vi "Build Simple Skeleton Data.vi"(8 "error in (no error)":errorcluster, 11 "connection ID":refnum<k16>) -> (0 "Kinect Outputs":T5, 1 "Skeleton Data":T6, 2 "NumPlayers":i8, 3 "Version String":string, 4 "Simple Joystick Info":T1(array[cluster]))   [LabVIEW 2013]
uses:
  <vilib>/addons/Kinect/SkeletonTrackState.ctl
  <vilib>/addons/Kinect/Vector4.ctl
  <vilib>/Rock Robotics/WPI/Joystick/WPI_JoystickDeviceDataRaw.ctl
  <vilib>/Rock Robotics/WPI/Dashboard/WPI_DashboardLogging Global.vi
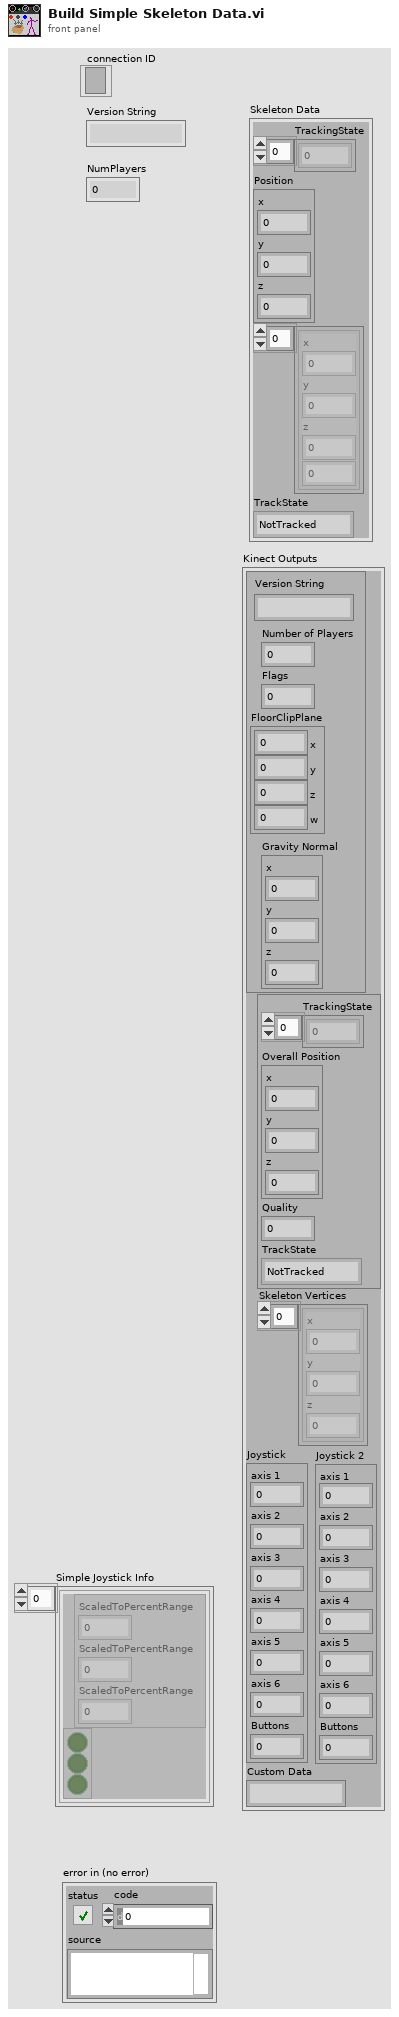
[diagram p1: front panel]
types:
  T1 = cluster{cluster{"ScaledToPercentRange":dbl, "ScaledToPercentRange":dbl, "ScaledToPercentRange":dbl}, cluster{bool, bool, bool}}[]
  T2 = typedef "Vector4.ctl" = cluster{"x":sgl, "y":sgl, "z":sgl, "w":sgl}
  T3 = typedef "SkeletonTrackState.ctl" = enum32{"NotTracked", "PositionOnly", "Tracked"}
  T4 = typedef "WPI_JoystickDeviceDataRaw.ctl" = cluster{"axis 1":i8, "axis 2":i8, "axis 3":i8, "axis 4":i8, "axis 5":i8, "axis 6":i8, "Buttons":u16}
  T5 = cluster{cluster{"Version String":string, "Number of Players":i8, "Flags":u32, "FloorClipPlane":T2, "Gravity Normal":cluster{"x":sgl, "y":sgl, "z":sgl}}, cluster{"TrackingState":u8[], "Overall Position":cluster{"x":sgl, "y":sgl, "z":sgl}, "Quality":u32, "TrackState":T3}, "Skeleton Vertices":cluster{"x":sgl, "y":sgl, "z":sgl}[], "Joystick":T4, "Joystick 2":T4, "Custom Data":string}
  T6 = cluster{"TrackingState":u8[], "Position":cluster{"x":sgl, "y":sgl, "z":sgl}, cluster{"x":sgl, "y":sgl, "z":sgl, sgl}[], "TrackState":T3}
  T7 = cluster{"size":u8, "tag":u8, "Version":cluster{"unsigned byte array[0]":u8, "unsigned byte array[1]":u8, "unsigned byte array[2]":u8, "unsigned byte array[3]":u8, "unsigned byte array[4]":u8, "unsigned byte array[5]":u8, "unsigned byte array[6]":u8, "unsigned byte array[7]":u8, "unsigned byte array[8]":u8, "unsigned byte array[9]":u8, "unsigned byte array[10]":u8}, "numPlayers":i8, "flags":u32, "floorClipPlane":T2, "Gravity Normal":cluster{"x":sgl, "y":sgl, "z":sgl}, "size":u8, "tag":u8, "Extra Data":cluster{"TrackingState":cluster{"TrackingState[0]":u8, "TrackingState[1]":u8, "TrackingState[2]":u8, "TrackingState[3]":u8, "TrackingState[4]":u8, "TrackingState[5]":u8, "TrackingState[6]":u8, "TrackingState[7]":u8, "TrackingState[8]":u8, "TrackingState[9]":u8, "TrackingState[10]":u8, "TrackingState[11]":u8, "TrackingState[12]":u8, "TrackingState[13]":u8, "TrackingState[14]":u8, "TrackingState[15]":u8, "TrackingState[16]":u8, "TrackingState[17]":u8, "TrackingState[18]":u8, "TrackingState[19]":u8}, "Position":cluster{"x":sgl, "y":sgl, "z":sgl}, "Quality":u32, "TrackState":T3}, "size":u8, "tag":u8, "Vertices":cluster{"Vertices[0]":cluster{"x":sgl, "y":sgl, "z":sgl}, "Vertices[1]":cluster{"x":sgl, "y":sgl, "z":sgl}, "Vertices[2]":cluster{"x":sgl, "y":sgl, "z":sgl}, "Vertices[3]":cluster{"x":sgl, "y":sgl, "z":sgl}, "Vertices[4]":cluster{"x":sgl, "y":sgl, "z":sgl}, "Vertices[5]":cluster{"x":sgl, "y":sgl, "z":sgl}, "Vertices[6]":cluster{"x":sgl, "y":sgl, "z":sgl}, "Vertices[7]":cluster{"x":sgl, "y":sgl, "z":sgl}, "Vertices[8]":cluster{"x":sgl, "y":sgl, "z":sgl}, "Vertices[9]":cluster{"x":sgl, "y":sgl, "z":sgl}, "Vertices[10]":cluster{"x":sgl, "y":sgl, "z":sgl}, "Vertices[11]":cluster{"x":sgl, "y":sgl, "z":sgl}, "Vertices[12]":cluster{"x":sgl, "y":sgl, "z":sgl}, "Vertices[13]":cluster{"x":sgl, "y":sgl, "z":sgl}, "Vertices[14]":cluster{"x":sgl, "y":sgl, "z":sgl}, "Vertices[15]":cluster{"x":sgl, "y":sgl, "z":sgl}, "Vertices[16]":cluster{"x":sgl, "y":sgl, "z":sgl}, "Vertices[17]":cluster{"x":sgl, "y":sgl, "z":sgl}, "Vertices[18]":cluster{"x":sgl, "y":sgl, "z":sgl}, "Vertices[19]":cluster{"x":sgl, "y":sgl, "z":sgl}}, "size":u8, "tag":u8, "Joystick":T4, "Joystick 2":T4, "size":u8, "tag":u8, "Custom Data":string}
  T8 = cluster{"size":u8, "tag":u8, "Version":cluster{"unsigned byte array[0]":u8, "unsigned byte array[1]":u8, "unsigned byte array[2]":u8, "unsigned byte array[3]":u8, "unsigned byte array[4]":u8, "unsigned byte array[5]":u8, "unsigned byte array[6]":u8, "unsigned byte array[7]":u8, "unsigned byte array[8]":u8, "unsigned byte array[9]":u8, "unsigned byte array[10]":u8}, "numPlayers":i8, "flags":u32, "floorClipPlane":T2, "Gravity Normal":cluster{"x":sgl, "y":sgl, "z":sgl}, "size":u8, "tag":u8, "Extra Data":cluster{"TrackingState":cluster{"TrackingState[0]":u8, "TrackingState[1]":u8, "TrackingState[2]":u8, "TrackingState[3]":u8, "TrackingState[4]":u8, "TrackingState[5]":u8, "TrackingState[6]":u8, "TrackingState[7]":u8, "TrackingState[8]":u8, "TrackingState[9]":u8, "TrackingState[10]":u8, "TrackingState[11]":u8, "TrackingState[12]":u8, "TrackingState[13]":u8, "TrackingState[14]":u8, "TrackingState[15]":u8, "TrackingState[16]":u8, "TrackingState[17]":u8, "TrackingState[18]":u8, "TrackingState[19]":u8}, "Position":cluster{"x":sgl, "y":sgl, "z":sgl}, "Quality":u32, "TrackState":T3}, "size":u8, "tag":u8, "Vertices":cluster{"Vertices[0]":cluster{"x":sgl, "y":sgl, "z":sgl}, "Vertices[1]":cluster{"x":sgl, "y":sgl, "z":sgl}, "Vertices[2]":cluster{"x":sgl, "y":sgl, "z":sgl}, "Vertices[3]":cluster{"x":sgl, "y":sgl, "z":sgl}, "Vertices[4]":cluster{"x":sgl, "y":sgl, "z":sgl}, "Vertices[5]":cluster{"x":sgl, "y":sgl, "z":sgl}, "Vertices[6]":cluster{"x":sgl, "y":sgl, "z":sgl}, "Vertices[7]":cluster{"x":sgl, "y":sgl, "z":sgl}, "Vertices[8]":cluster{"x":sgl, "y":sgl, "z":sgl}, "Vertices[9]":cluster{"x":sgl, "y":sgl, "z":sgl}, "Vertices[10]":cluster{"x":sgl, "y":sgl, "z":sgl}, "Vertices[11]":cluster{"x":sgl, "y":sgl, "z":sgl}, "Vertices[12]":cluster{"x":sgl, "y":sgl, "z":sgl}, "Vertices[13]":cluster{"x":sgl, "y":sgl, "z":sgl}, "Vertices[14]":cluster{"x":sgl, "y":sgl, "z":sgl}, "Vertices[15]":cluster{"x":sgl, "y":sgl, "z":sgl}, "Vertices[16]":cluster{"x":sgl, "y":sgl, "z":sgl}, "Vertices[17]":cluster{"x":sgl, "y":sgl, "z":sgl}, "Vertices[18]":cluster{"x":sgl, "y":sgl, "z":sgl}, "Vertices[19]":cluster{"x":sgl, "y":sgl, "z":sgl}}, "size":u8, "tag":u8, "Joystick":T4, "Joystick 2":T4, "size":u8, "tag":u8, "Custom Data":string}[]
  T9 = cluster{"unsigned byte array[0]":u8, "unsigned byte array[1]":u8, "unsigned byte array[2]":u8, "unsigned byte array[3]":u8, "unsigned byte array[4]":u8, "unsigned byte array[5]":u8, "unsigned byte array[6]":u8, "unsigned byte array[7]":u8, "unsigned byte array[8]":u8, "unsigned byte array[9]":u8, "unsigned byte array[10]":u8}
  T10 = cluster{"TrackingState[0]":u8, "TrackingState[1]":u8, "TrackingState[2]":u8, "TrackingState[3]":u8, "TrackingState[4]":u8, "TrackingState[5]":u8, "TrackingState[6]":u8, "TrackingState[7]":u8, "TrackingState[8]":u8, "TrackingState[9]":u8, "TrackingState[10]":u8, "TrackingState[11]":u8, "TrackingState[12]":u8, "TrackingState[13]":u8, "TrackingState[14]":u8, "TrackingState[15]":u8, "TrackingState[16]":u8, "TrackingState[17]":u8, "TrackingState[18]":u8, "TrackingState[19]":u8}
  T11 = cluster{"Vertices[0]":cluster{"x":sgl, "y":sgl, "z":sgl}, "Vertices[1]":cluster{"x":sgl, "y":sgl, "z":sgl}, "Vertices[2]":cluster{"x":sgl, "y":sgl, "z":sgl}, "Vertices[3]":cluster{"x":sgl, "y":sgl, "z":sgl}, "Vertices[4]":cluster{"x":sgl, "y":sgl, "z":sgl}, "Vertices[5]":cluster{"x":sgl, "y":sgl, "z":sgl}, "Vertices[6]":cluster{"x":sgl, "y":sgl, "z":sgl}, "Vertices[7]":cluster{"x":sgl, "y":sgl, "z":sgl}, "Vertices[8]":cluster{"x":sgl, "y":sgl, "z":sgl}, "Vertices[9]":cluster{"x":sgl, "y":sgl, "z":sgl}, "Vertices[10]":cluster{"x":sgl, "y":sgl, "z":sgl}, "Vertices[11]":cluster{"x":sgl, "y":sgl, "z":sgl}, "Vertices[12]":cluster{"x":sgl, "y":sgl, "z":sgl}, "Vertices[13]":cluster{"x":sgl, "y":sgl, "z":sgl}, "Vertices[14]":cluster{"x":sgl, "y":sgl, "z":sgl}, "Vertices[15]":cluster{"x":sgl, "y":sgl, "z":sgl}, "Vertices[16]":cluster{"x":sgl, "y":sgl, "z":sgl}, "Vertices[17]":cluster{"x":sgl, "y":sgl, "z":sgl}, "Vertices[18]":cluster{"x":sgl, "y":sgl, "z":sgl}, "Vertices[19]":cluster{"x":sgl, "y":sgl, "z":sgl}}
  T12 = cluster{"TrackingState":cluster{"TrackingState[0]":u8, "TrackingState[1]":u8, "TrackingState[2]":u8, "TrackingState[3]":u8, "TrackingState[4]":u8, "TrackingState[5]":u8, "TrackingState[6]":u8, "TrackingState[7]":u8, "TrackingState[8]":u8, "TrackingState[9]":u8, "TrackingState[10]":u8, "TrackingState[11]":u8, "TrackingState[12]":u8, "TrackingState[13]":u8, "TrackingState[14]":u8, "TrackingState[15]":u8, "TrackingState[16]":u8, "TrackingState[17]":u8, "TrackingState[18]":u8, "TrackingState[19]":u8}, "Position":cluster{"x":sgl, "y":sgl, "z":sgl}, "Quality":u32, "TrackState":T3}
  T13 = cluster{"ScaledToPercentRange":dbl, "ScaledToPercentRange":dbl, "ScaledToPercentRange":dbl}
  T14 = cluster{cluster{"ScaledToPercentRange":dbl, "ScaledToPercentRange":dbl, "ScaledToPercentRange":dbl}, cluster{bool, bool, bool}}
  T15 = cluster{"string":string, "numPlayers":i8, "flags":u32, "floorClipPlane":T2, "Gravity Normal":cluster{"x":sgl, "y":sgl, "z":sgl}}
  T16 = cluster{"TrackingState":u8[], "Position":cluster{"x":sgl, "y":sgl, "z":sgl}, "Quality":u32, "TrackState":T3}
  T17 = cluster{cluster{"string":string, "numPlayers":i8, "flags":u32, "floorClipPlane":T2, "Gravity Normal":cluster{"x":sgl, "y":sgl, "z":sgl}}, cluster{"TrackingState":u8[], "Position":cluster{"x":sgl, "y":sgl, "z":sgl}, "Quality":u32, "TrackState":T3}, "Vertices":cluster{"x":sgl, "y":sgl, "z":sgl}[], "Joystick":T4, "Joystick 2":T4, "Custom Data":string}
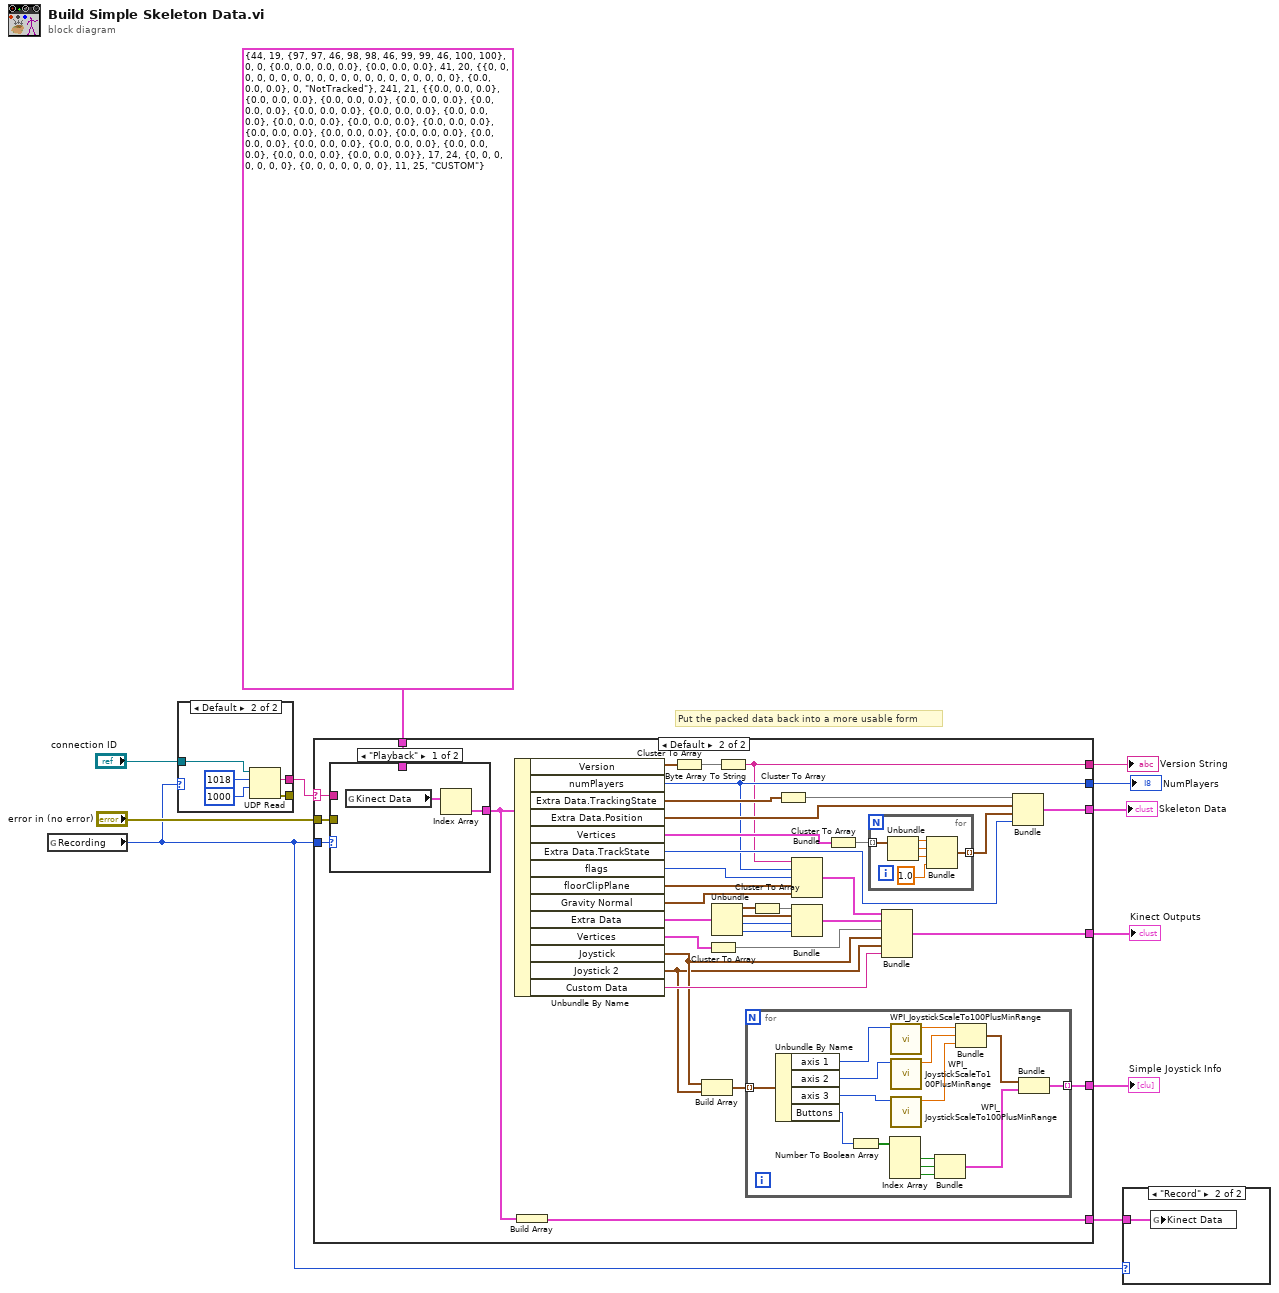
[diagram p0: block diagram]
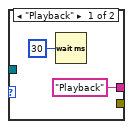
[diagram p3: hidden frame]
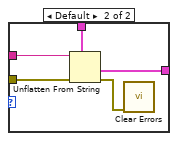
[diagram p5: hidden frame]
diagram:
  # "Put the packed data back into a more usable form"
  n1 = global read "WPI_DashboardLogging Global.vi" "Recording"() -> (w1:enum32{"Stop", "Record", "Playback"})
  n2 = case shown="Default" w1 {
    tunnel: ["Playback" ("data out") w16] -> w3
    tunnel: "connection ID" -> [_ w15]
    tunnel: [_ w14] -> _
    frame "Playback" {
      n3 = Wait (ms)(milliseconds to wait=u32 30) -> ()  [unwired: 1 out]
    }
    frame Default {
      n4 = UDP Read(connection ID=w15, max size (548)=1018 ("bytes to read"), timeout ms (25000)=1000) -> (data out=w16:string, error out=w14:errorcluster)  [unwired: 1 in, 3 out]
    }
  }
  n5 = case shown="Default" w3 {
    selector: w3 -> [_ w22]
    tunnel: [_ w49] -> w11
    tunnel: T7 {"size"=44, "tag"=19, "Version"={"unsigned byte array[0]"=97, "unsigned byte array[1]"=97, "unsigned byte array[2]"=46, "unsigned byte array[3]"=98, "unsigned byte array[4]"=98, "unsigned byte array[5]"=46, "unsigned byte array[6]"=99, "unsigned byte array[7]"=99, "unsigned byte array[8]"=46, "unsigned byte array[9]"=100, "unsigned byte array[10]"=100}, "numPlayers"=0, "flags"=0, "floorClipPlane"={"x"=0.0, "y"=0.0, "z"=0.0, "w"=0.0}, "Gravity Normal"={"x"=0.0, "y"=0.0, "z"=0.0}, "size"=41, "tag"=20, "Extra Data"={"TrackingState"={"TrackingState[0]"=0, "TrackingState[1]"=0, "TrackingState[2]"=0, "TrackingState[3]"=0, "TrackingState[4]"=0, "TrackingState[5]"=0, "TrackingState[6]"=0, "TrackingState[7]"=0, "TrackingState[8]"=0, "TrackingState[9]"=0, "TrackingState[10]"=0, "TrackingState[11]"=0, "TrackingState[12]"=0, "TrackingState[13]"=0, "TrackingState[14]"=0, "TrackingState[15]"=0, "TrackingState[16]"=0, "TrackingState[17]"=0, "TrackingState[18]"=0, "TrackingState[19]"=0}, "Position"={"x"=0.0, "y"=0.0, "z"=0.0}, "Quality"=0, "TrackState"=enum."NotTracked"}, "size"=241, "tag"=21, "Vertices"={"Vertices[0]"={"x"=0.0, "y"=0.0, "z"=0.0}, "Vertices[1]"={"x"=0.0, "y"=0.0, "z"=0.0}, "Vertices[2]"={"x"=0.0, "y"=0.0, "z"=0.0}, "Vertices[3]"={"x"=0.0, "y"=0.0, "z"=0.0}, "Vertices[4]"={"x"=0.0, "y"=0.0, "z"=0.0}, "Vertices[5]"={"x"=0.0, "y"=0.0, "z"=0.0}, "Vertices[6]"={"x"=0.0, "y"=0.0, "z"=0.0}, "Vertices[7]"={"x"=0.0, "y"=0.0, "z"=0.0}, "Vertices[8]"={"x"=0.0, "y"=0.0, "z"=0.0}, "Vertices[9]"={"x"=0.0, "y"=0.0, "z"=0.0}, "Vertices[10]"={"x"=0.0, "y"=0.0, "z"=0.0}, "Vertices[11]"={"x"=0.0, "y"=0.0, "z"=0.0}, "Vertices[12]"={"x"=0.0, "y"=0.0, "z"=0.0}, "Vertices[13]"={"x"=0.0, "y"=0.0, "z"=0.0}, "Vertices[14]"={"x"=0.0, "y"=0.0, "z"=0.0}, "Vertices[15]"={"x"=0.0, "y"=0.0, "z"=0.0}, "Vertices[16]"={"x"=0.0, "y"=0.0, "z"=0.0}, "Vertices[17]"={"x"=0.0, "y"=0.0, "z"=0.0}, "Vertices[18]"={"x"=0.0, "y"=0.0, "z"=0.0}, "Vertices[19]"={"x"=0.0, "y"=0.0, "z"=0.0}}, "size"=17, "tag"=24, "Joystick"={"axis 1"=0, "axis 2"=0, "axis 3"=0, "axis 4"=0, "axis 5"=0, "axis 6"=0, "Buttons"=0}, "Joystick 2"={"axis 1"=0, "axis 2"=0, "axis 3"=0, "axis 4"=0, "axis 5"=0, "axis 6"=0, "Buttons"=0}, "size"=11, "tag"=25, "Custom Data"="CUSTOM"} ("output data") -> [_ w46]
    tunnel: [_ w44] -> w9
    tunnel: [_ w30] -> w8
    tunnel: [_ w29] -> w7
    tunnel: [_ w24] -> w6
    tunnel: "error in (no error)" -> [_ w23]
    tunnel: [_ w20] -> w4
    tunnel: w1 -> [_ w19]
    frame "" {
    }
    frame Default {
      n6 = case shown="\"Playback\"" w19 {
        tunnel: w46 -> [_ w62]
        tunnel: w23 -> [_ w60]
        tunnel: w22 -> [_ w59]
        tunnel: [w56 w58] -> w21
        frame "Playback" {
          n7 = global read "WPI_DashboardLogging Global.vi" "Kinect Data"() -> (w57:T8)
          n8 = Index Array(array=w57) -> (element=w56:T7)  [unwired: 1 in]
        }
        frame Default {
          n9 = Unflatten From String(type=w62, binary string=w59, error in (no error)=w60) -> (value=w58:T7, error out=w61:errorcluster)  [unwired: 3 out]
          n10 = call <vilib>:"Clear Errors.vi"("error in (no error)"=w61) -> ()  [unwired: 6 in, 1 out]
        }
      }
      n11 = Unbundle By Name(w21) -> ("Version"=w45:T9, "numPlayers"=w44:i8, "Extra Data.TrackingState"=w48:T10, "Extra Data.Position"=w54:cluster{"x":sgl, "y":sgl, "z":sgl}, "Vertices"=w53:T11, "Extra Data.TrackState"=w55:T3, "flags"=w43:u32, "floorClipPlane"=w42:T2, "Gravity Normal"=w41:cluster{"x":sgl, "y":sgl, "z":sgl}, "Extra Data"=w39:T12, "Vertices"=w32:T11, "Joystick"=w27:T4, "Joystick 2"=w25:T4, "Custom Data"=w28:string)
      n12 = Build Array(w21) -> (w20:T8)
      n13 = Cluster To Array(cluster=w45) -> (array=w47:u8[])
      n14 = Build Array(w27, w25) -> (w26:T4[])
      n15 = Cluster To Array(cluster=w32) -> (array=w31:cluster{"x":sgl, "y":sgl, "z":sgl}[])
      n16 = Unbundle(w39) -> ("TrackingState"=w38:T10, "Position"=w36:cluster{"x":sgl, "y":sgl, "z":sgl}, "Quality"=w35:u32, "TrackState"=w34:T3)
      n17 = Byte Array To String(unsigned byte array=w47) -> (string=w29:string)
      n18 = for {
        tunnel: w26 -> [w77] mode=indexing
        tunnel: [w63] -> w24 mode=indexing
        n19 = Unbundle By Name(w77) -> ("axis 1"=w71:i8, "axis 2"=w69:i8, "axis 3"=w68:i8, "Buttons"=w75:u16)
        n20 = Number To Boolean Array(number=w75) -> (Boolean array=w76:bool[])
        n21 = Index Array(array=w76) -> (element #1=w72:bool, element #2=w73:bool, element #3=w74:bool)  [unwired: 3 in]
        n22 = call <vilib>:"WPI_JoystickScaleTo100PlusMinRange.vi"("RawValue"=w71) -> ("ScaledToPercentRange"=w70:dbl)  [unwired: 1 in, 9 out]
        n23 = call <vilib>:"WPI_JoystickScaleTo100PlusMinRange.vi"("RawValue"=w69) -> ("ScaledToPercentRange"=w67:dbl)  [unwired: 1 in, 9 out]
        n24 = call <vilib>:"WPI_JoystickScaleTo100PlusMinRange.vi"("RawValue"=w68) -> ("ScaledToPercentRange"=w66:dbl)  [unwired: 1 in, 9 out]
        n25 = Bundle(w72, w73, w74) -> (w64:cluster{bool, bool, bool})  [unwired: 1 in]
        n26 = Bundle("ScaledToPercentRange"=w70, "ScaledToPercentRange"=w67, "ScaledToPercentRange"=w66) -> (w65:T13)  [unwired: 1 in]
        n27 = Bundle(w65, w64) -> (w63:T14)  [unwired: 1 in]
      }
      n28 = Cluster To Array(cluster=w38) -> (array=w37:u8[])
      n29 = Cluster To Array(cluster=w48) -> (array=w50:u8[])
      n30 = Bundle("string"=w29, "numPlayers"=w44, "flags"=w43, "floorClipPlane"=w42, "Gravity Normal"=w41) -> (w40:T15)  [unwired: 1 in]
      n31 = Bundle("TrackingState"=w37, "Position"=w36, "Quality"=w35, "TrackState"=w34) -> (w33:T16)  [unwired: 1 in]
      n32 = Cluster To Array(cluster=w53) -> (array=w51:cluster{"x":sgl, "y":sgl, "z":sgl}[])
      n33 = for {
        tunnel: w51 -> [w83] mode=indexing
        tunnel: [w78] -> w52 mode=indexing
        n34 = Unbundle(w83) -> ("x"=w79:sgl, "y"=w80:sgl, "z"=w81:sgl)
        n35 = Bundle("x"=w79, "y"=w80, "z"=w81, sgl 1.0) -> (w78:cluster{"x":sgl, "y":sgl, "z":sgl, sgl})  [unwired: 1 in]
      }
      n36 = Bundle(w40, w33, "Vertices"=w31, "Joystick"=w27, "Joystick 2"=w25, "Custom Data"=w28) -> (w30:T17)  [unwired: 1 in]
      n37 = Bundle("TrackingState"=w50, "Position"=w54, w52, "TrackState"=w55) -> (w49:T6)  [unwired: 1 in]
    }
  }
  "Skeleton Data" <- w11
  "NumPlayers" <- w9
  "Version String" <- w7
  "Kinect Outputs" <- w8
  "Simple Joystick Info" <- w6
  n38 = case shown="\"Record\"" w1 {
    tunnel: w4 -> [_ w84]
    frame Default {
    }
    frame "Record" {
      n39 = global write "WPI_DashboardLogging Global.vi" "Kinect Data"(w84) -> ()
    }
  }
